vi "UTIL Predict Class Multivariate HMM.vi"(5 "Data Point":dbl[](array[numeric]), 8 "Model Information":dbl[][](array[numeric]), 9 "d(t-1) In":dbl[](array[numeric])) -> (2 "Sleep Stage":i32, 3 "d(t-1) Out":dbl[](array[numeric]))   [LabVIEW 2017]
doc: "This VI approximates the current sleep state given a data point using a Hidden Markov Model. Each state cluster is represented as amultivariate gaussian distribution with vector mean mu and covariance matrix sigma. The VI keeps track of current and previous probabilities and takes into acount the transition probabilities between states to determine the current state, approximating the forward portion of the Viterbi Algorithm.\n\nInputs:\n Data Point 1D Array of DBL, Current data point\n in 3D feature space\n Model Information 2D Array of DBL,MATLAB computed \n centroids covariance matrices, priors, \n and transition matrix\n d(t-1) In Delta from previous time point to be used in Viterbi Algorithm\n\nOutputs:\n Sleep Stage SGL, assigned sleep stage prediction\n d(t-1) Out Delta to be used in next iteration"
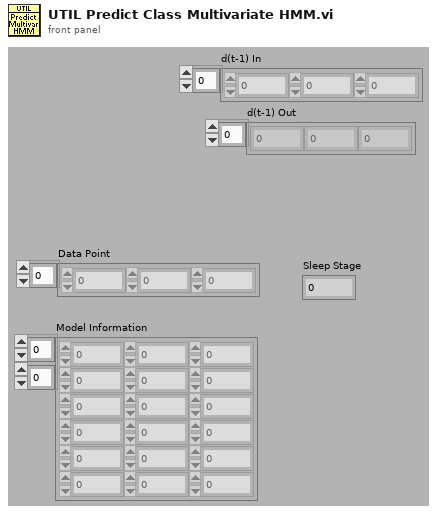
[diagram p1: front panel]
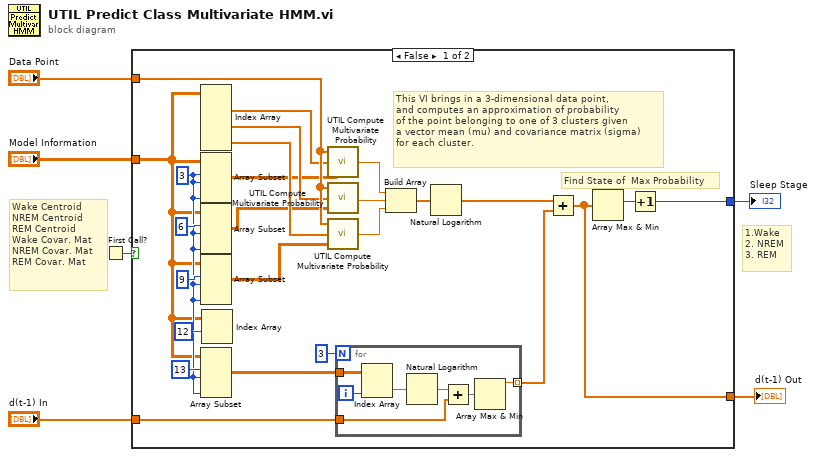
[diagram p0: block diagram]
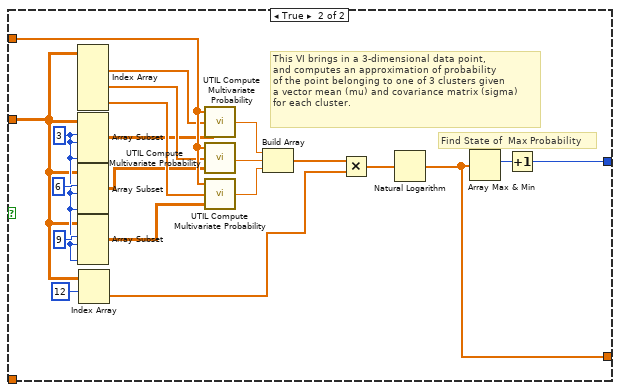
[diagram p2: hidden frame]
diagram:
  # "Wake Centroid\nNREM Centroid\nREM Centroid\nWake Covar. Mat\nNREM Covar. Mat\nREM Covar. Mat"
  # "1.Wake\n2. NREM\n3. REM"
  n1 = First Call?() -> (First Call?: T/F=w1:bool)
  n2 = case shown="False" w1 {
    tunnel: [w31 w59] -> w6
    tunnel: "Data Point" -> [w24 w55]
    tunnel: "Model Information" -> [w9 w43]
    tunnel: "d(t-1) In" -> [w29 _]
    tunnel: [w28 w39] -> w2
    frame False {
      w10 = 3 ("index")
      # "This VI brings in a 3-dimensional data point,\nand computes an approximation of probability\nof the point belonging to one of 3 clusters given \na vector mean (mu) and covariance matrix (sigma)\nfor each cluster."
      # "Find State of  Max Probability"
      n3 = Index Array(array=w9) -> (element #1=w23:dbl[], element #2=w22:dbl[], element #3=w21:dbl[])  [unwired: 6 in]
      n4 = Array Subset(array=w9, index (row)=w10, length (row)=w10, length (col)=w10) -> (w20:dbl[][])  [unwired: 1 in]
      n5 = Array Subset(array=w9, index (row)=6 ("index"), length (row)=w10, length (col)=w10) -> (w19:dbl[][])  [unwired: 1 in]
      n6 = Array Subset(array=w9, index (row)=9 ("index"), length (row)=w10, length (col)=w10) -> (w13:dbl[][])  [unwired: 1 in]
      n7 = Array Subset(array=w9, index (row)=13 ("index"), length (row)=w10, length (col)=w10) -> (w8:dbl[][])  [unwired: 1 in]
      n8 = Index Array(array=w9, index (row)=12) -> ()  [unwired: 1 in, 1 out]
      n9 = call "UTIL Compute Multivariate Probability.vi"("Sigma"=w20, "Mu"=w23, "Data Point"=w24) -> ("P(x,mu,sigma)"=w18:dbl)  [unwired: 2 in]
      n10 = call "UTIL Compute Multivariate Probability.vi"("Sigma"=w19, "Mu"=w22, "Data Point"=w24) -> ("P(x,mu,sigma)"=w17:dbl)  [unwired: 2 in]
      n11 = call "UTIL Compute Multivariate Probability.vi"("Sigma"=w13, "Mu"=w21, "Data Point"=w24) -> ("P(x,mu,sigma)"=w16:dbl)  [unwired: 2 in]
      n12 = for {
        N: 3 ("Numeric") -> [_]
        tunnel: w8 -> [w37]
        tunnel: w29 -> [w38]
        tunnel: [w34] -> w14 mode=indexing
        i -> [w32]
        n13 = Index Array(array=w37, index (col)=w32) -> (element=w36:dbl[])  [unwired: 1 in]
        n14 = Natural Logarithm(1:w36) -> (0:w33:dbl[])
        n15 = Add(x=w33, y=w38) -> (x+y=w35:dbl[])
        n16 = Array Max & Min(array=w35) -> (max value=w34:dbl)  [unwired: 3 out]
      }
      n17 = Build Array(w18, w17, w16) -> (w15:dbl[])
      n18 = Natural Logarithm(1:w15) -> (0:w7:dbl[])
      n19 = Add(x=w7, y=w14) -> (x+y=w28:dbl[])
      n20 = Array Max & Min(array=w28) -> (max index (indices)=w30:i32)  [unwired: 3 out]
      n21 = Increment(x=w30) -> (x+1=w31:i32)
    }
    frame True {
      w44 = 3 ("index")
      # "This VI brings in a 3-dimensional data point,\nand computes an approximation of probability\nof the point belonging to one of 3 clusters given \na vector mean (mu) and covariance matrix (sigma)\nfor each cluster."
      # "Find State of  Max Probability"
      n22 = Index Array(array=w43) -> (element #1=w54:dbl[], element #2=w53:dbl[], element #3=w52:dbl[])  [unwired: 6 in]
      n23 = Array Subset(array=w43, index (row)=w44, length (row)=w44, length (col)=w44) -> (w51:dbl[][])  [unwired: 1 in]
      n24 = Array Subset(array=w43, index (row)=6 ("index"), length (row)=w44, length (col)=w44) -> (w50:dbl[][])  [unwired: 1 in]
      n25 = Array Subset(array=w43, index (row)=9 ("index"), length (row)=w44, length (col)=w44) -> (w46:dbl[][])  [unwired: 1 in]
      n26 = Index Array(array=w43, index (row)=12) -> (element=w40:dbl[])  [unwired: 1 in]
      n27 = call "UTIL Compute Multivariate Probability.vi"("Sigma"=w51, "Mu"=w54, "Data Point"=w55) -> ("P(x,mu,sigma)"=w49:dbl)  [unwired: 2 in]
      n28 = call "UTIL Compute Multivariate Probability.vi"("Sigma"=w50, "Mu"=w53, "Data Point"=w55) -> ("P(x,mu,sigma)"=w48:dbl)  [unwired: 2 in]
      n29 = call "UTIL Compute Multivariate Probability.vi"("Sigma"=w46, "Mu"=w52, "Data Point"=w55) -> ("P(x,mu,sigma)"=w47:dbl)  [unwired: 2 in]
      n30 = Build Array(w49, w48, w47) -> (w41:dbl[])
      n31 = Multiply(x=w41, y=w40) -> (x*y=w42:dbl[])
      n32 = Natural Logarithm(1:w42) -> (0:w39:dbl[])
      n33 = Array Max & Min(array=w39) -> (max index (indices)=w58:i32)  [unwired: 3 out]
      n34 = Increment(x=w58) -> (x+1=w59:i32)
    }
  }
  "Sleep Stage" <- w6
  "d(t-1) Out" <- w2
